vi "State Enter Core.vi"(8 "error in":errorcluster, 11 "A State in":refnum<class "A State.lvclass">) -> (0 "error out":errorcluster, 3 "A State out":refnum<class "A State.lvclass">)   [LabVIEW 2021, in "Context.lvlib" / "A State.lvclass"]
uses:
  A State.lvclass
  A State.lvclass/A State.ctl
  Context/Context.lvclass
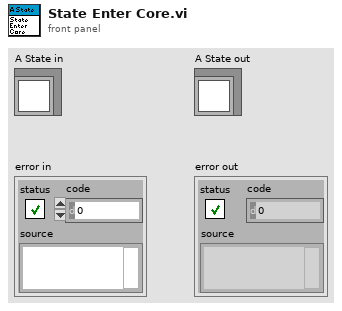
[diagram p1: front panel]
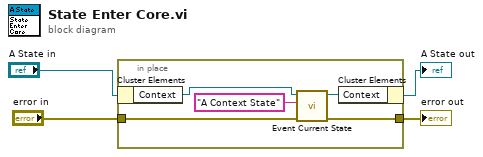
[diagram p0: block diagram]
diagram:
  n1 = in-place {
    in-place-border: "error in" -> [w7]
    in-place-border: [w6] -> w1
    n2 = in-place-cluster #1("A State in") -> ("Context"=w9:refnum<class "Context.lvclass">)
    n3 = call "Event Current State.vi"("error in"=w7, "Current State"="A Context State", "Context in"=w9) -> ("error out"=w6:errorcluster, "Context out"=w8:refnum<class "Context.lvclass">)  [unwired: 7 in]
    n4 = in-place-cluster #1("Context"=w8) -> (→"A State out":refnum<class "A State.lvclass">)
  }
  "error out" <- w1
